vi "Limit switch.vi"(11 "Enum":enum16{"Start", "Run", "End"}(ring)) -> (3 "Value":bool)   [LabVIEW 2012]
uses:
  TypeDefs/Digital Module 1.ctl
  <vilib>/Rock Robotics/SystemInterfaces/Typedef/FPGA_TypedefDigitalModule.ctl
  <vilib>/Rock Robotics/SystemInterfaces/DIO/FPGA_DIOChannel.ctl
panel:
  in  "Digital Module A":T1={"Module"=enum."Digital Module 1", "Unassigned"=enum."DIO 1", "Unassigned"=enum."DIO 2", "Unassigned"=enum."DIO 3", "Unassigned"=enum."DIO 4", "Unassigned"=enum."DIO 5", "Unassigned"=enum."DIO 6", "Unassigned"=enum."DIO 7", "Unassigned"=enum."DIO 8", "Unassigned"=enum."DIO 9", "Unassigned"=enum."DIO 10", "Unassigned"=enum."DIO 11", "Unassigned"=enum."DIO 12", "Unassigned"=enum."DIO 13", "Unassigned"=enum."DIO 14"}
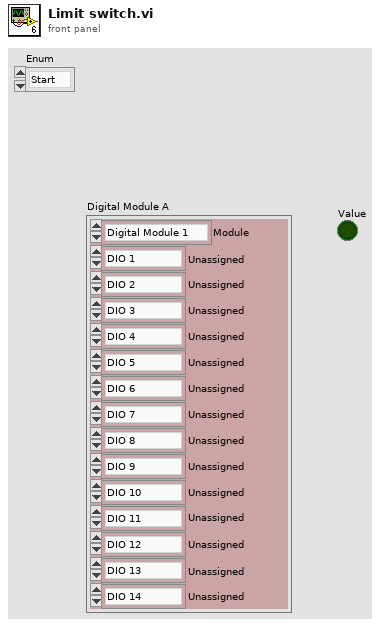
[diagram p1: front panel]
types:
  T1 = typedef "Digital Module 1.ctl" = cluster{"Module":T2, "Unassigned":T3, "Unassigned":T3, "Unassigned":T3, "Unassigned":T3, "Unassigned":T3, "Unassigned":T3, "Unassigned":T3, "Unassigned":T3, "Unassigned":T3, "Unassigned":T3, "Unassigned":T3, "Unassigned":T3, "Unassigned":T3, "Unassigned":T3}
  T2 = typedef "FPGA_TypedefDigitalModule.ctl" = enum16{"Digital Module 1", "Digital Module 2"}
  T3 = typedef "FPGA_DIOChannel.ctl" = enum8{"DIO 1", "DIO 2", "DIO 3", "DIO 4", "DIO 5", "DIO 6", "DIO 7", "DIO 8", "DIO 9", "DIO 10", "DIO 11", "DIO 12", "DIO 13", "DIO 14", "Invalid"}
  T4 = typedef "WPI_DigitalInputDevRef.ctl" = cluster{"DevStatus":errorcluster, "DIO Channel":T3, "Digital Module":T2}
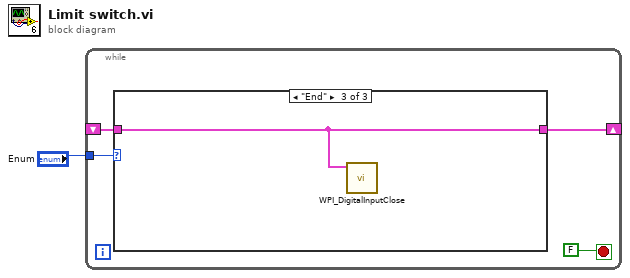
[diagram p0: block diagram]
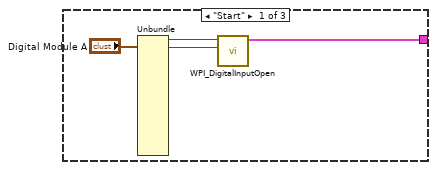
[diagram p2: hidden frame]
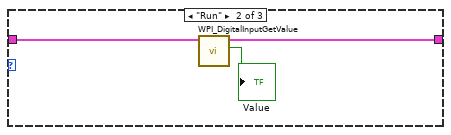
[diagram p3: hidden frame]
diagram:
  n1 = while {
    shift-right: [w5] -> _
    shift-left: _ -> [w4]
    tunnel: "Enum" -> [w2]
    stop <- FALSE ("stop") stop-if-true
    n2 = case shown="\"End\"" w2 {
      tunnel: [w9 w11 w13] -> w5
      tunnel: w4 -> [_ w12 w13]
      frame "Start" {
        n3 = Unbundle("Digital Module A") -> ("Module"=w7:T2, "Unassigned"=w6:T3)  [unwired: 13 out]
        n4 = call <vilib>:"WPI_DigitalInputOpen.vi"("DIO Channel"=w6, "Digital Module (Module 1)"=w7) -> ("DigitalInputDevRef"=w9:T4)  [unwired: 8 in, 1 out]
      }
      frame "Run" {
        n5 = call <vilib>:"WPI_DigitalInputGetValue.vi"("DigitalInputDevRef"=w12) -> ("Value"=→"Value":bool, "DigitalInputDevRef"=w11:T4)  [unwired: 8 in, 1 out]
      }
      frame "End" {
        n6 = call <vilib>:"WPI_DigitalInputClose.vi"("DigitalInputDevRef"=w13) -> ()  [unwired: 10 in, 1 out]
      }
    }
  }
